vi "Logic-CheckSelectData.vi"(8 "error in (no error)":errorcluster, 11 "TableLogger Config":T1) -> (0 "error out":errorcluster)   [LabVIEW 2014, in "TableLogger_SQLite_Actor.lvlib" / "TableLogger_SQLite_Actor.lvclass"]
uses:
  TableLogger_SQLite_Actor.lvclass
  TableLogger_Actor/TableLoggerConfig.ctl
  TableLogger_Actor/TableLoggerTypes.ctl
  TableLogger_Actor/TableLoggerBackupConfig.ctl
  TableLogger_Actor/TableLogger_Actor.lvlib
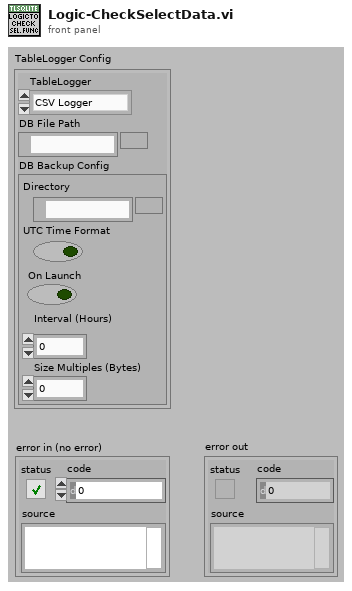
[diagram p1: front panel]
types:
  T1 = typedef "TableLogger_Actor.lvlib/TableLoggerConfig.ctl" = cluster{"TableLogger":T2, "DB File Path":path, "DB Backup Config":T3}
  T2 = typedef "TableLogger_Actor.lvlib/TableLoggerTypes.ctl" = enum16{"CSV Logger", "SQLite Logger"}
  T3 = typedef "TableLogger_Actor.lvlib/TableLoggerBackupConfig.ctl" = cluster{"Directory":path, "UTC Time Format":bool, "On Launch":bool, "Interval (Hours)":dbl, "Size Multiples (Bytes)":i32}
  T4 = cluster{"Numeric Data":i32, "Float Data":dbl, "String Data":string, "Enum Data":enum16{"Enum Item 1", "Enum Item 2"}, "Array Data":i32[], "Array Data 2":i32[], "Numeric Data 2":i32, "Array Data 3":i32[]}[]
  T5 = cluster{"Numeric Data":i32, "Float Data":dbl, "String Data":string, "Enum Data":enum16{"Enum Item 1", "Enum Item 2"}, "Array Data":i32[]}
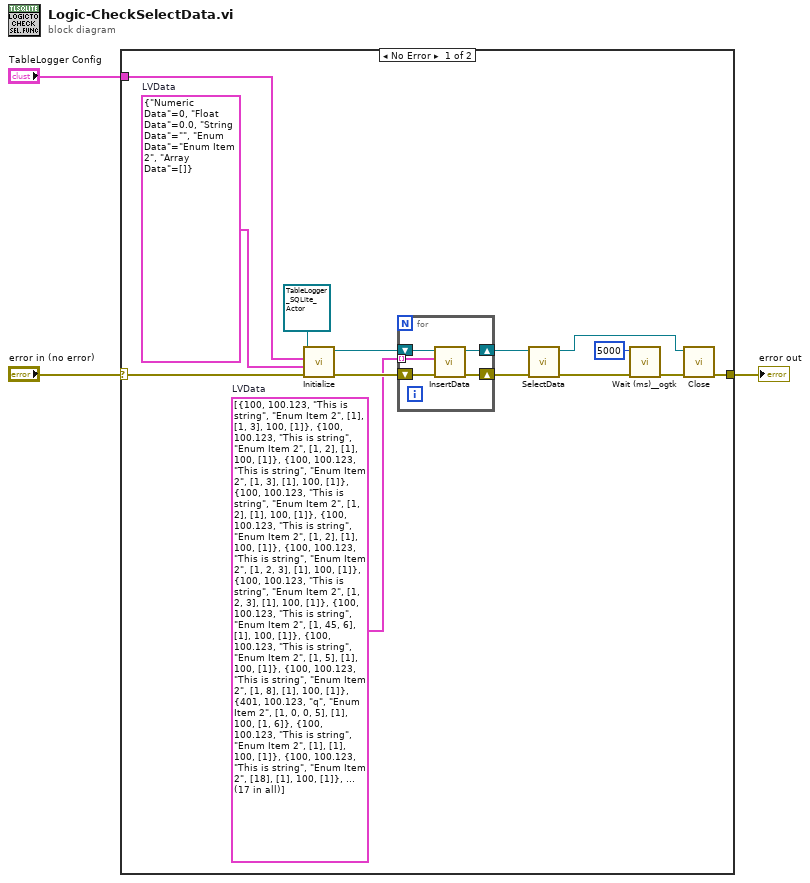
[diagram p0: block diagram]
diagram:
  n1 = case shown="No Error" "error in (no error)" {
    selector: "error in (no error)" -> [w16 w23]
    tunnel: "TableLogger Config" -> [w5 _]
    tunnel: [w4 w23] -> w1
    frame No Error {
      w10 = T4 [{"Numeric Data"=100, "Float Data"=100.123, "String Data"="This is string", "Enum Data"=enum."Enum Item 2", "Array Data"=[1], "Array Data 2"=[1, 3], "Numeric Data 2"=100, "Array Data 3"=[1]}, {"Numeric Data"=100, "Float Data"=100.123, "String Data"="This is string", "Enum Data"=enum."Enum Item 2", "Array Data"=[1, 2], "Array Data 2"=[1], "Numeric Data 2"=100, "Array Data 3"=[1]}, {"Numeric Data"=100, "Float Data"=100.123, "String Data"="This is string", "Enum Data"=enum."Enum Item 2", "Array Data"=[1, 3], "Array Data 2"=[1], "Numeric Data 2"=100, "Array Data 3"=[1]}, {"Numeric Data"=100, "Float Data"=100.123, "String Data"="This is string", "Enum Data"=enum."Enum Item 2", "Array Data"=[1, 2], "Array Data 2"=[1], "Numeric Data 2"=100, "Array Data 3"=[1]}, {"Numeric Data"=100, "Float Data"=100.123, "String Data"="This is string", "Enum Data"=enum."Enum Item 2", "Array Data"=[1, 2], "Array Data 2"=[1], "Numeric Data 2"=100, "Array Data 3"=[1]}, {"Numeric Data"=100, "Float Data"=100.123, "String Data"="This is string", "Enum Data"=enum."Enum Item 2", "Array Data"=[1, 2, 3], "Array Data 2"=[1], "Numeric Data 2"=100, "Array Data 3"=[1]}, {"Numeric Data"=100, "Float Data"=100.123, "String Data"="This is string", "Enum Data"=enum."Enum Item 2", "Array Data"=[1, 2, 3], "Array Data 2"=[1], "Numeric Data 2"=100, "Array Data 3"=[1]}, {"Numeric Data"=100, "Float Data"=100.123, "String Data"="This is string", "Enum Data"=enum."Enum Item 2", "Array Data"=[1, 45, 6], "Array Data 2"=[1], "Numeric Data 2"=100, "Array Data 3"=[1]}, {"Numeric Data"=100, "Float Data"=100.123, "String Data"="This is string", "Enum Data"=enum."Enum Item 2", "Array Data"=[1, 5], "Array Data 2"=[1], "Numeric Data 2"=100, "Array Data 3"=[1]}, {"Numeric Data"=100, "Float Data"=100.123, "String Data"="This is string", "Enum Data"=enum."Enum Item 2", "Array Data"=[1, 8], "Array Data 2"=[1], "Numeric Data 2"=100, "Array Data 3"=[1]}, {"Numeric Data"=401, "Float Data"=100.123, "String Data"="q", "Enum Data"=enum."Enum Item 2", "Array Data"=[1, 0, 0, 5], "Array Data 2"=[1], "Numeric Data 2"=100, "Array Data 3"=[1, 6]}, {"Numeric Data"=100, "Float Data"=100.123, "String Data"="This is string", "Enum Data"=enum."Enum Item 2", "Array Data"=[1], "Array Data 2"=[1], "Numeric Data 2"=100, "Array Data 3"=[1]}, {"Numeric Data"=100, "Float Data"=100.123, "String Data"="This is string", "Enum Data"=enum."Enum Item 2", "Array Data"=[18], "Array Data 2"=[1], "Numeric Data 2"=100, "Array Data 3"=[1]}, {"Numeric Data"=100, "Float Data"=100.123, "String Data"="This is string", "Enum Data"=enum."Enum Item 2", "Array Data"=[1, 0, 0, 0, 98], "Array Data 2"=[1], "Numeric Data 2"=100, "Array Data 3"=[1]}, {"Numeric Data"=100, "Float Data"=100.123, "String Data"="This is string", "Enum Data"=enum."Enum Item 2", "Array Data"=[1, 2], "Array Data 2"=[1, 2], "Numeric Data 2"=100, "Array Data 3"=[1]}, {"Numeric Data"=100, "Float Data"=100.123, "String Data"="This is string", "Enum Data"=enum."Enum Item 2", "Array Data"=[1, 2, 2], "Array Data 2"=[1], "Numeric Data 2"=100, "Array Data 3"=[1]}, {"Numeric Data"=100, "Float Data"=100.123, "String Data"="This is string", "Enum Data"=enum."Enum Item 2", "Array Data"=[1], "Array Data 2"=[1, 1], "Numeric Data 2"=100, "Array Data 3"=[1]}]  # LVData
      w7 = T5 {"Numeric Data"=0, "Float Data"=0.0, "String Data"="", "Enum Data"=enum."Enum Item 2", "Array Data"=[]}  # LVData
      n2 = call-dynamic "Initialize.vi"("error in (no error)"=w16, "Data Cluster (for Table Headers)"=w7, "TableLogger Config"=w5, "object in"=refnum<class "TableLogger_SQLite_Actor.lvclass"> refnum) -> ("error out"=w13:errorcluster, "object out"=w11:refnum<class "TableLogger_SQLite_Actor.lvclass">)  [unwired: 6 in]
      n3 = for {
        shift-right: [w21] -> w14
        shift-left: w13 -> [w22]
        shift-right: [w19] -> w12
        shift-left: w11 -> [w20]
        tunnel: w10 -> [w18] mode=indexing
        n4 = call-dynamic "InsertData.vi"("error in (no error)"=w22, "Data Cluster"=w18, "object in"=w20) -> ("error out"=w21:errorcluster, "object out"=w19:refnum<class "TableLogger_SQLite_Actor.lvclass">)  [unwired: 7 in]
      }
      n5 = call-dynamic "SelectData.vi"("error in (no error)"=w14, "object in"=w12) -> ("error out"=w17:errorcluster, "object out"=w15:refnum<class "TableLogger_SQLite_Actor.lvclass">)  [unwired: 7 in, 1 out]
      n6 = call <userlib>:"Wait (ms)__ogtk.vi"("error in (no error)"=w17, "milliseconds to wait"=u32 5000) -> ("error out"=w8:errorcluster)  [unwired: 8 in, 1 out]
      n7 = call-dynamic "Close.vi"("error in (no error)"=w8, "object in"=w15) -> ("error out"=w4:errorcluster)  [unwired: 8 in, 1 out]
    }
    frame Error {
    }
  }
  "error out" <- w1
